vi "I2C_Stop.vi"(5 "TransmitDelay(Ticks)":u32, 7 "HalfCycle(Ticks)":u32, 8 "error in":errorcluster) -> (0 "error out":errorcluster)   [LabVIEW 2019]
doc: "Sends a STOP out the I2C Bus\n\n<b>Inputs:</b>\n---------------------\n<b>HalfCycle(Ticks)</b> this the number of FPGA clock cycles in half og the clock period. Therefore twice this number yields the clock period, in ticks.\n\n<b>TransmitDelay(Ticks)</b> the delay in FPGA clock cycles before writing bytes on SDA.\n---------------------\nSee block diagram for more details on the implementation details.\n\nAuthor:\nPeter Fuller\nSenior Engineer\nPLF Consulting, LLC\n\nemail: peter@plfconsulting.com\nphone: 617.699.2201"
uses:
  <vilib>/eio/EIONode/EIONode.xnode
  Instance           4 16Saved   I2C_Stop .vi
  Instance           5 16Saved   I2C_Stop .vi
  Instance           1 16Saved   I2C_Stop .vi
  <vilib>/eio/EIOMethodNode/EIOMethodNode.xnode
  <vilib>/rvi/eio/common/nirviEmuTemplateMethod_errors.vi
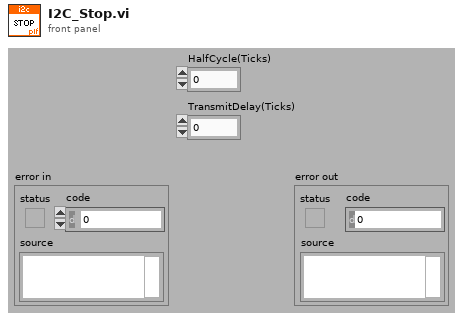
[diagram p1: front panel]
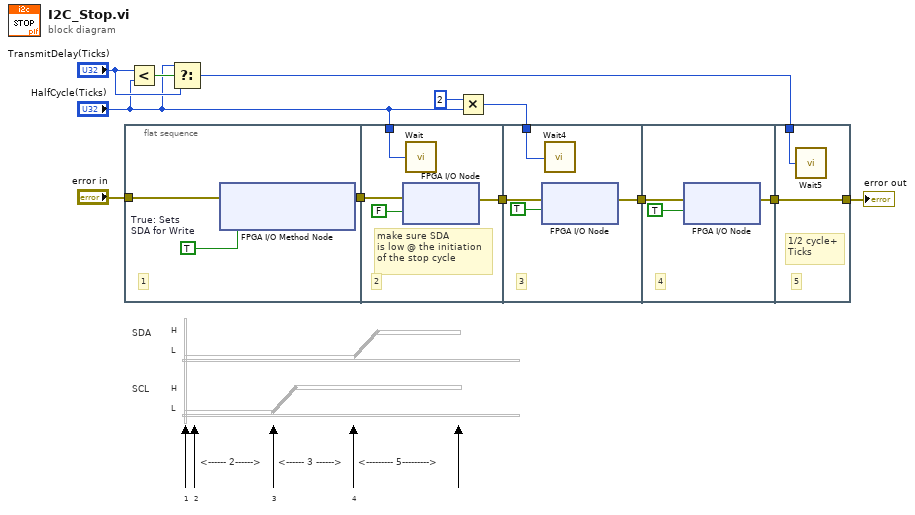
[diagram p0: block diagram]
diagram:
  # "<--------- 5--------->"
  # "<------ 3 ------>"
  # "2"
  # "H\n\nL"
  # "H\n\nL"
  # "4"
  # "<------ 2------>"
  # "3"
  # "1"
  # "SCL"
  # "SDA"
  n1 = flat-sequence {
    tunnel: "error in" -> [w14]
    tunnel: [w13] -> w7
    tunnel: w7 -> [w18]
    tunnel: [w17] -> w5
    tunnel: "HalfCycle(Ticks)" -> [w16]
    tunnel: w5 -> [w22]
    tunnel: [w21] -> w3
    tunnel: w4 -> [w20]
    tunnel: w3 -> [w25]
    tunnel: [w24] -> w1
    tunnel: w10 -> [w28]
    tunnel: [w27] -> w2
    tunnel: w1 -> [w27]
    frame #0 {
      w15 = TRUE  # True: Sets  SDA for Write
      # "1"
      n2 = xnode "FPGA I/O Method Node"("error in"=w14, "Enable"=w15) -> ("error out"=w13:errorcluster)  [unwired: 1 in, 1 out]
    }
    frame #1 {
      # "2"
      # "make sure SDA\nis low @ the initiation\nof the stop cycle"
      n3 = xnode "FPGA I/O Node"("error in"=w18, "SDA"=FALSE ("Value")) -> ("error out"=w17:errorcluster)  [unwired: 1 in, 1 out]
      n4 = call "Wait"("Count(Ticks)"=w16) -> ()  [unwired: 1 out]
    }
    frame #2 {
      # "3"
      n5 = xnode "FPGA I/O Node"("error in"=w22, "SCL"=TRUE ("Value")) -> ("error out"=w21:errorcluster)  [unwired: 1 in, 1 out]
      n6 = call "Wait4"("Count(Ticks)"=w20) -> ()  [unwired: 1 out]
    }
    frame #3 {
      # "4"
      n7 = xnode "FPGA I/O Node"("error in"=w25, "SDA"=TRUE ("Value")) -> ("error out"=w24:errorcluster)  [unwired: 1 in, 1 out]
    }
    frame #4 {
      # "5"
      # "1/2 cycle+\nTicks"
      n8 = call "Wait5"("Count(Ticks)"=w28) -> ()  [unwired: 1 out]
    }
  }
  n9 = Less?(x="TransmitDelay(Ticks)", y="HalfCycle(Ticks)") -> (x < y?=w12:bool)
  n10 = Select(t="HalfCycle(Ticks)", s=w12, f="TransmitDelay(Ticks)") -> (s? t:f=w10:u32)
  n11 = Multiply(x=u32 2, y="HalfCycle(Ticks)") -> (x*y=w4:u32)
  "error out" <- w2
